vi "Material-ProcessResults-WriteDb.vi"(8 "error in (no error)":errorcluster, 11 "Material-RunTest in":refnum<class "Material-RunTest.lvclass">) -> (0 "error out":errorcluster, 3 "Material-RunTest out":refnum<class "Material-RunTest.lvclass">)   [LabVIEW 2013, in "Material-RunTest.lvclass"]
uses:
  Material-RunTest.lvclass
  Material-RunTest.lvclass/Material-RunTest.ctl
  Reuse Library/Database API/Database-API.lvclass
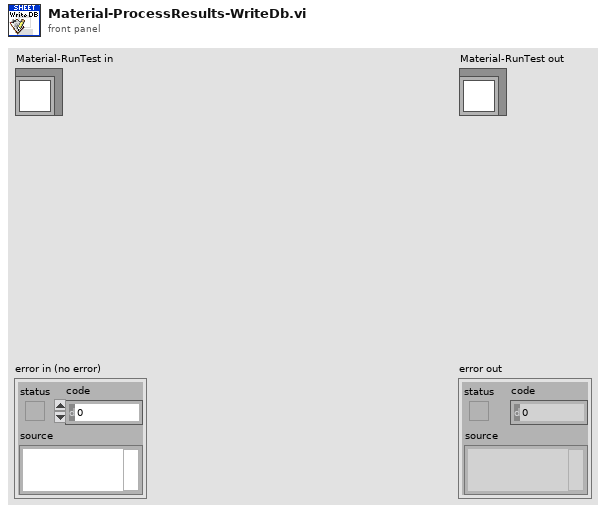
[diagram p1: front panel]
types:
  T1 = cluster{"Lot Number":string, "Line 1 AVG":dbl, "Line 2 AVG":dbl, "Line 3 AVG":dbl, "Value":dbl, string}
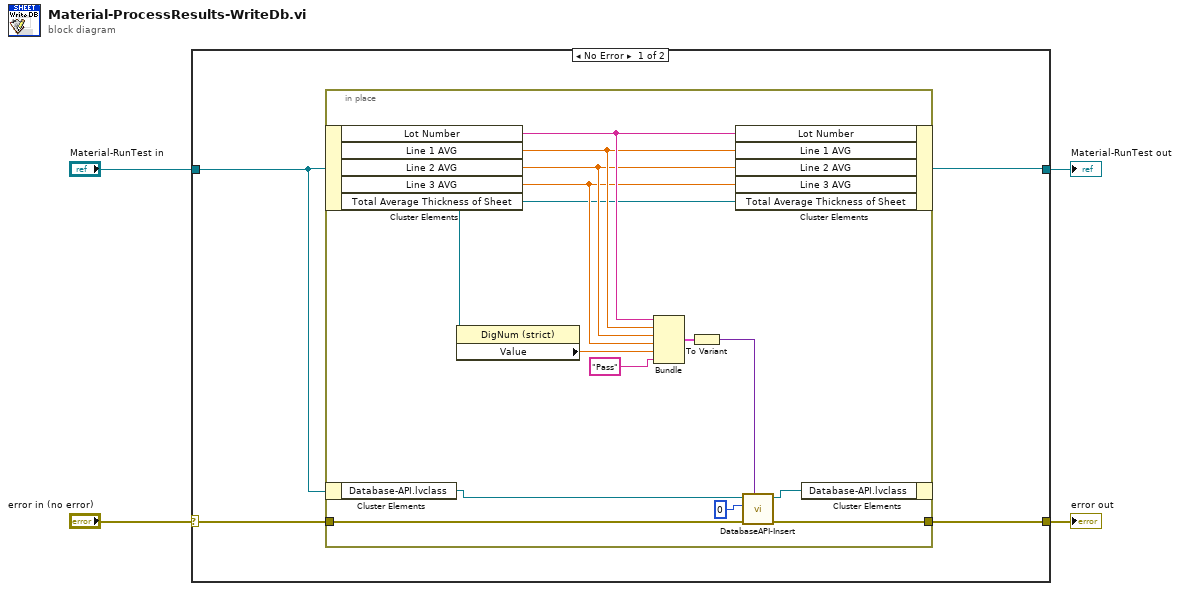
[diagram p0: block diagram]
diagram:
  n1 = case shown="No Error" "error in (no error)" {
    selector: "error in (no error)" -> [w8 w24]
    tunnel: [w6 w24] -> w3
    tunnel: [w5 w23] -> w1
    tunnel: "Material-RunTest in" -> [w7 w23]
    frame No Error {
      n2 = in-place {
        in-place-border: w8 -> [w22]
        in-place-border: [w9] -> w6
        n3 = in-place-cluster #1(w7) -> ("Lot Number"=w17:string, "Line 1 AVG"=w16:dbl, "Line 2 AVG"=w15:dbl, "Line 3 AVG"=w14:dbl, "Total Average Thickness of Sheet"=w13:refnum<vi>)
        n4 = in-place-cluster #2(w7) -> ("Database-API.lvclass"=w21:refnum<class "Database-API.lvclass">)
        n5 = property class="DigNum (strict)"(reference=w13) -> ("Value"=w19:dbl)  [unwired: 1 in, 2 out]
        n6 = Bundle("Lot Number"=w17, "Line 1 AVG"=w16, "Line 2 AVG"=w15, "Line 3 AVG"=w14, "Value"=w19, "Pass") -> (w12:T1)  [unwired: 1 in]
        n7 = To Variant(anything=w12) -> (Variant=w11:variant)
        n8 = in-place-cluster #1("Lot Number"=w17, "Line 1 AVG"=w16, "Line 2 AVG"=w15, "Line 3 AVG"=w14, "Total Average Thickness of Sheet"=w13) -> (w5:refnum<class "Material-RunTest.lvclass">)
        n9 = call "DatabaseAPI-Insert.vi"("Cluster Data for DB"=w11, "error in (no error)"=w22, "Table"=0, "Database-API in"=w21) -> ("error out"=w9:errorcluster, "Database-API out"=w10:refnum<class "Database-API.lvclass">)  [unwired: 6 in]
        n10 = in-place-cluster #2("Database-API.lvclass"=w10) -> ()  [unwired: 1 out]
      }
    }
    frame Error {
    }
  }
  "error out" <- w3
  "Material-RunTest out" <- w1
